vi "(TestVI)DW7802 PWL Graph Annotation Test.vi"() -> ()   [LabVIEW 2020]
uses:
  <vilib>/Utility/miscctls.llb/LVAnnotationListTypeDef.ctl
panel:
  out "x*y":dbl
  out "클래스 이름":string
  out "커서 인덱스":i32
  out "커서 위치":cluster{"X":dbl, "Y":dbl}
  in  "정지":bool
  in  "주석 리스트 2":T1=[{"Name"="p0", "Color"=16711680, "Style"=0, "Point Style"=6, "Name Visible"=TRUE, "Allow Drag"=TRUE, "Annotation Mode"=0, "Plot"=-1, "Index"=0, "Position"={"X"=50.0, "Y"=0.0}, "X Scale"=0, "Y Scale"=0, "Show Arrow"=FALSE, "Lock Name"=FALSE, "Plot Area"=0, "Label Offset"={"X"=0.0, "Y"=1.0}}, {"Name"="p1", "Color"=16711680, "Style"=0, "Point Style"=6, "Name Visible"=TRUE, "Allow Drag"=TRUE, "Annotation Mode"=0, "Plot"=-1, "Index"=0, "Position"={"X"=60.0, "Y"=0.0}, "X Scale"=0, "Y Scale"=0, "Show Arrow"=FALSE, "Lock Name"=FALSE, "Plot Area"=0, "Label Offset"={"X"=0.0, "Y"=1.0}}, {"Name"="p2", "Color"=16711680, "Style"=0, "Point Style"=6, "Name Visible"=TRUE, "Allow Drag"=TRUE, "Annotation Mode"=0, "Plot"=-1, "Index"=0, "Position"={"X"=70.0, "Y"=0.0}, "X Scale"=0, "Y Scale"=0, "Show Arrow"=FALSE, "Lock Name"=FALSE, "Plot Area"=0, "Label Offset"={"X"=0.0, "Y"=1.0}}] caption="주석 리스트" {"Color" format="%06x"}
  out "주석 리스트":T1
  out "웨이브폼 그래프":dbl[](graph)
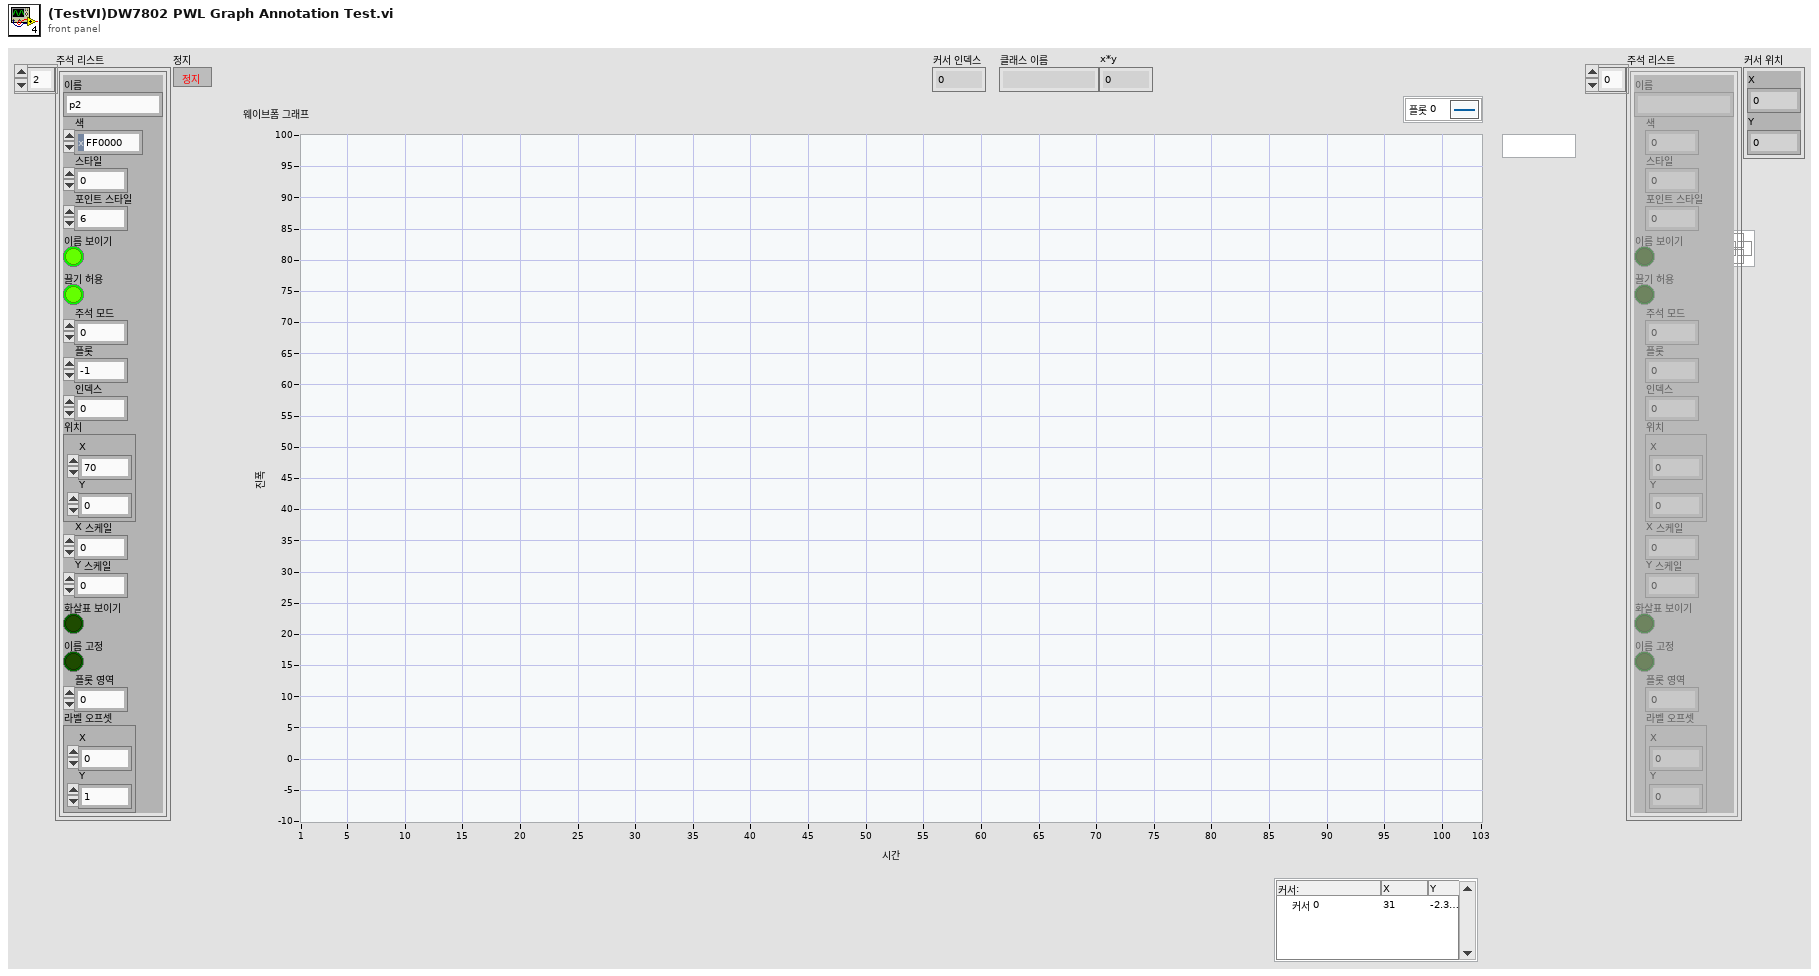
[diagram p1: front panel]
types:
  T1 = typedef "LVAnnotationListTypeDef.ctl" = cluster{"Name":string, "Color":u32, "Style":u8, "Point Style":u8, "Name Visible":bool, "Allow Drag":bool, "Annotation Mode":u32, "Plot":i32, "Index":i32, "Position":cluster{"X":dbl, "Y":dbl}, "X Scale":u32, "Y Scale":u32, "Show Arrow":bool, "Lock Name":bool, "Plot Area":i32, "Label Offset":cluster{"X":dbl, "Y":dbl}}[]
  T2 = cluster{"Name":string, "Color":u32, "Style":u8, "Point Style":u8, "Name Visible":bool, "Allow Drag":bool, "Annotation Mode":u32, "Plot":i32, "Index":i32, "Position":cluster{"X":dbl, "Y":dbl}, "X Scale":u32, "Y Scale":u32, "Show Arrow":bool, "Lock Name":bool, "Plot Area":i32, "Label Offset":cluster{"X":dbl, "Y":dbl}}
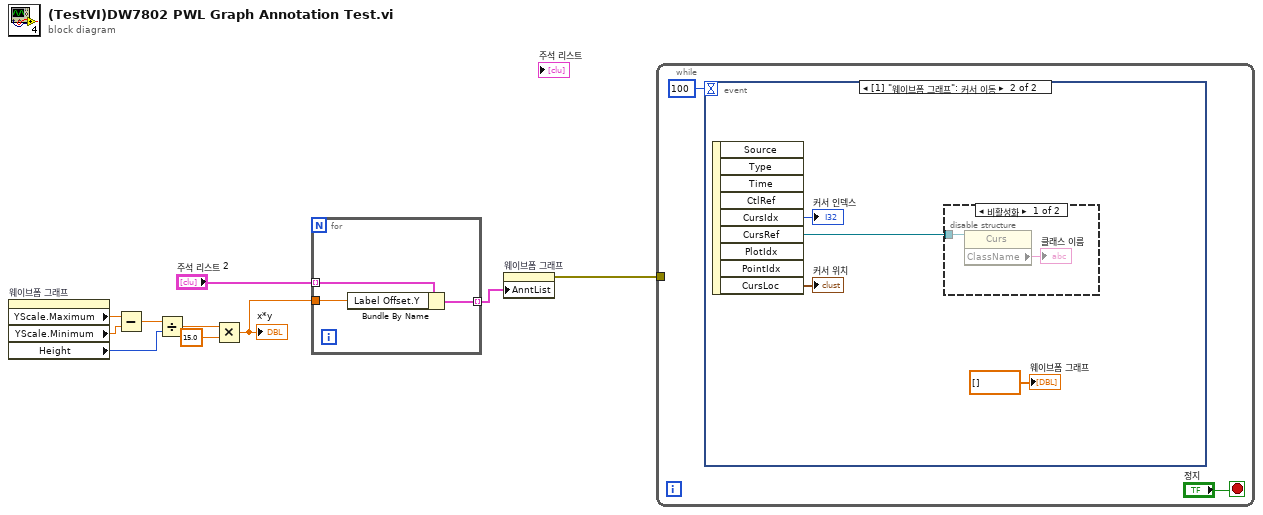
[diagram p0: block diagram]
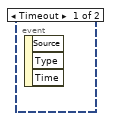
[diagram p2: hidden frame]
diagram:
  n1 = property on="웨이브폼 그래프" class="WFGraph (엄격한)"() -> ("YScale.Maximum"=w10:dbl, "YScale.Minimum"=w9:dbl, "Height"=w7:u32)  [unwired: 2 in, 2 out]
  n2 = Subtract(x=w10, y=w9) -> (x-y=w8:dbl)
  n3 = Divide(x=w8, y=w7) -> (x/y=w6:dbl)
  n4 = Multiply(x=w6, y=15.0) -> (x*y=w3:dbl)
  "x*y" <- w3
  n5 = for {
    tunnel: "주석 리스트 2" -> [w13] mode=indexing
    tunnel: w3 -> [w12]
    tunnel: [w11] -> w2 mode=indexing
    n6 = Bundle By Name(cluster=w13, "Label Offset.Y"=w12) -> (w11:T2)
  }
  n7 = property on="웨이브폼 그래프" class="WFGraph (엄격한)"("AnntList"=w2) -> (error out=w1:errorcluster)  [unwired: 2 in, 1 out]
  n8 = while {
    tunnel: w1 -> [_]
    stop <- "정지" stop-if-true
    n9 = event shown="[1] \"웨이브폼 그래프\": 커서 이동" {
      selector: _ -> [_ _]
      dyn-events: _ -> [_ _]
      timeout: 100 -> [_ _]
      event Timeout {
        n10 = event-data() -> ()  [unwired: 1 in, 3 out]
      }
      event "웨이브폼 그래프": Cursor Move {
        n11 = event-data() -> ("CursIdx"=→"커서 인덱스":i32, "CursRef"=w16:refnum<vi>, "CursLoc"=→"커서 위치":cluster{"X":dbl, "Y":dbl})  [unwired: 1 in, 6 out]
        n12 = disable-structure shown="비활성화" {
          disable-tunnel: w16 -> [w20 _]
          frame Disabled {
            n13 = property class="Curs"(reference=w20) -> ("ClassName"=→"클래스 이름":string)  [unwired: 1 in, 2 out]
          }
          frame Enabled {
          }
        }
        "웨이브폼 그래프" <- dbl[] [] ("웨이브폼 그래프")
      }
    }
  }
